vi "RDS Child Core Init.vi"(8 "error in (no error)":errorcluster, 11 "RDS Parent Actor in":refnum<class "RDS Parent Actor.lvclass">) -> (0 "error out":errorcluster, 1 "RDS Router Enqeuer":refnum<class "Message Enqueuer.lvclass">, 2 "Event Registration Refnum":refnum<event-registration>, 3 "RDS Parent Actor out":refnum<class "RDS Parent Actor.lvclass">)   [LabVIEW 2015, in "RDS Abstracts.lvlib" / "RDS Parent Actor.lvlib" / "RDS Parent Actor.lvclass"]
uses:
  RDS Parent Actor.lvclass
  <vilib>/ActorFramework/Message Enqueuer/Message Enqueuer.lvclass
  RDS Parent Actor.lvclass/RDS Parent Actor.ctl
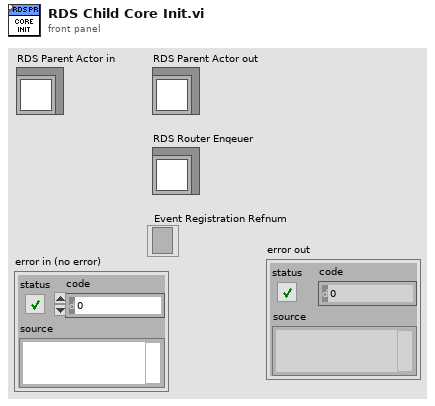
[diagram p1: front panel]
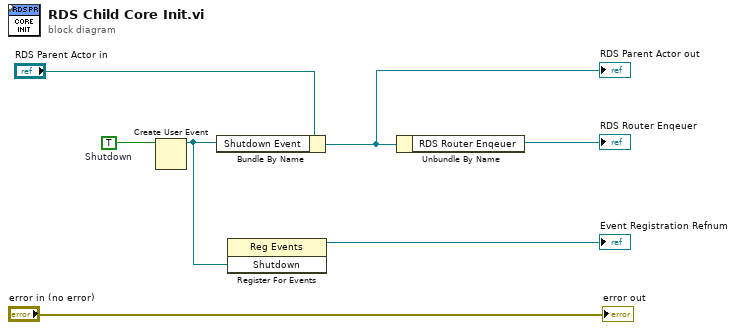
[diagram p0: block diagram]
diagram:
  w2 = TRUE  # Shutdown
  n1 = Create User Event(user event datatype=w2) -> (user event=w3:refnum<user-event>)  [unwired: 1 in, 1 out]
  n2 = Bundle By Name(cluster="RDS Parent Actor in", "Shutdown Event"=w3) -> (w6:refnum<class "RDS Parent Actor.lvclass">)
  "RDS Parent Actor out" <- w6
  n3 = register-events(w3) -> (reference out=→"Event Registration Refnum":refnum<event-registration>)  [unwired: 2 in, 1 out]
  n4 = Unbundle By Name(w6) -> ("RDS Router Enqeuer"=→"RDS Router Enqeuer":refnum<class "Message Enqueuer.lvclass">)
  "error out" <- "error in (no error)"
